vi "2023 Process Arm Reach Spreadsheet.vi"(1 "error in":errorcluster, 2 "armReachSpreadSheet":string[][](array[string])) -> (0 "error out":errorcluster)   [LabVIEW 2020]
uses:
  2023 Input Arm To Wrist Global.vi
panel:
  out "inputToArmToWristConversion":dbl[](array[numeric])
  out "element 2":string
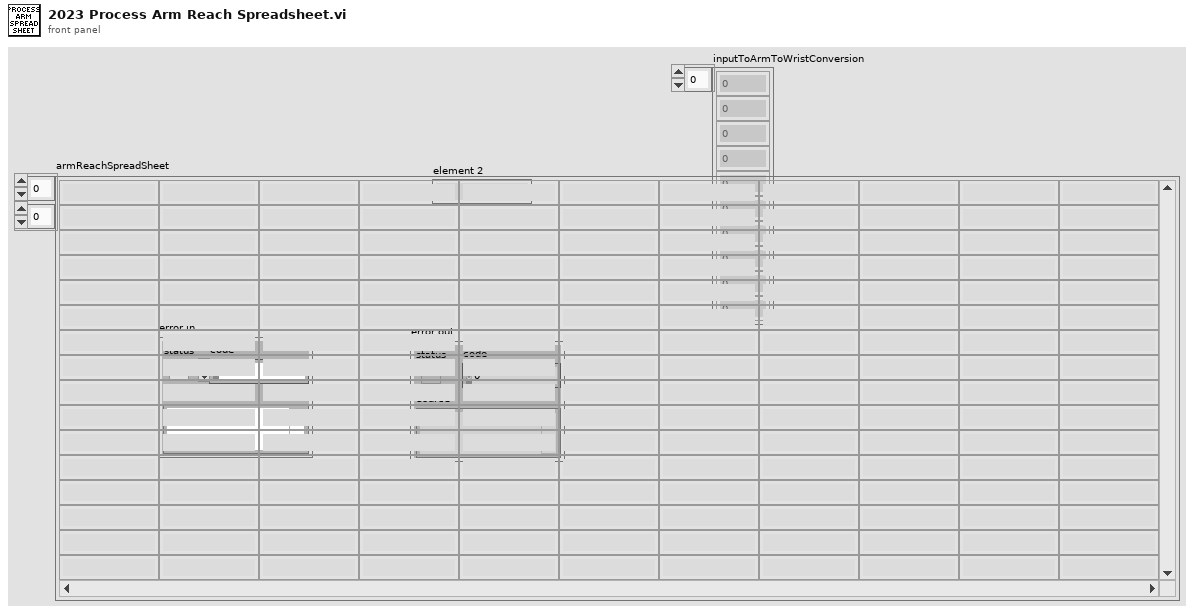
[diagram p1: front panel]
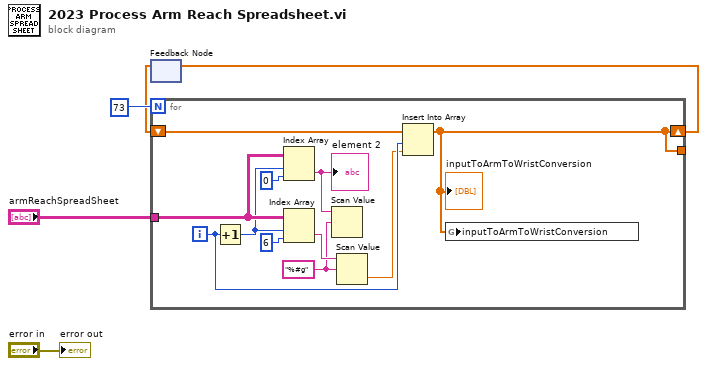
[diagram p0: block diagram]
diagram:
  n1 = feedback #1() -> (w3:dbl[])  [unwired: 1 in]
  n2 = for {
    N: 73 -> [_]
    tunnel: "armReachSpreadSheet" -> [w14]
    shift-right: [w6] -> w4
    shift-left: w3 -> [w7]
    tunnel: [w6] -> _
    i -> [w9]
    w10 = "%#g" ("format string")
    n3 = Increment(x=w9) -> (x+1=w13:i32)
    n4 = Index Array(array=w14, index (row)=w13, index (col)=0 ("disabled index (col)")) -> (element=w15:string)
    "element 2" <- w15
    n5 = Index Array(array=w14, index (row)=w13, index (col)=6 ("disabled index (col)")) -> (element=w11:string)
    n6 = Scan Value(string=w15, format string=w10) -> ()  [unwired: 1 in, 2 out]
    n7 = Scan Value(string=w11, format string=w10) -> (value=w8:dbl)  [unwired: 1 in, 1 out]
    n8 = Insert Into Array(array=w7, index=w9, new element=w8) -> (w6:dbl[])
    "inputToArmToWristConversion" <- w6
    n9 = global write "2023 Input Arm To Wrist Global.vi" "inputToArmToWristConversion"(w6) -> ()
  }
  n10 = feedback-in #1(w4) -> ()
  "error out" <- "error in"
